vi "Agilent SNA Read Measurement.vi"(6 "Channel":i8=1 min=1 max=99 step=1, 7 "Agilent SNA & SWP":T2, 8 "error in (no error)":errorcluster, 11 "VISA Resource Names":T3) -> (0 "error out":errorcluster, 1 "Parameter":T1 {"Stimulus Port" min=1 step=1; "Response Port" min=1 step=1}, 2 "Measurement":T4=enum."Analog In - Aux In", 3 "dup VISA Resource Names":T3)   [LabVIEW 2011]
doc: "This VI for the HP 8753B is used to read the meausurement format.\n\n0 log magnitude\n1 phase\n2 delay\n3 Smith chart\n4 polar\n5 linear magnitude\n6 standing wave ratio\n7 real\n8 imaginary"
uses:
  TypeDefs/Agilent SNA Measurement.ctl
  TypeDefs/Agilent SNA VISA.ctl
  TypeDefs/Agilent SNA Instrument Info.ctl
  tests/S Parameter/TypeDefs/SP Parameter.ctl
panel:
  in  "Trace":i8=1 min=1 max=99 step=1
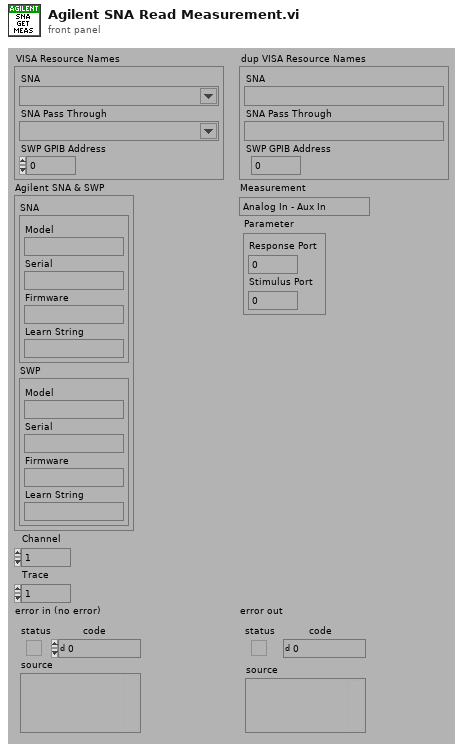
[diagram p1: front panel]
types:
  T1 = typedef "SP Parameter.ctl" = cluster{"Stimulus Port":i8, "Response Port":i8}
  T2 = typedef "Agilent SNA Instrument Info.ctl" = cluster{"SNA":cluster{"Model":string, "Serial":string, "Firmware":string, "Learn String":string}, "SWP":cluster{"Model":string, "Serial":string, "Firmware":string, "Learn String":string}}
  T3 = typedef "Agilent SNA VISA.ctl" = cluster{"SNA":refnum<visa-resource-name>, "SNA Pass Through":refnum<visa-resource-name>, "SWP GPIB Address":i32}
  T4 = typedef "Agilent SNA Measurement.ctl" = enum32{"SXX", "A", "B", "C", "R", "A/B", "A/C", "A/R", "B/A", "B/C", "B/R", "C/A", "C/B", "C/R", "R/A", "R/B", "R/C", "Analog In - Aux In"}
  T5 = typedef "Agilent SNA Model.ctl" = enum16{"Not Supported", "8757X"}
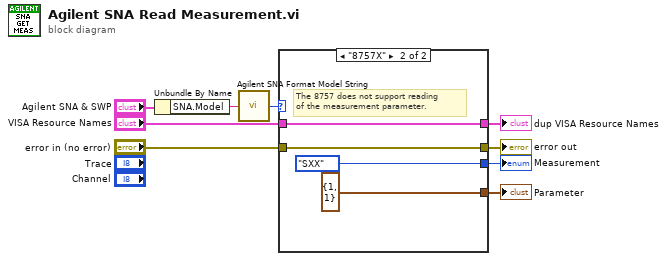
[diagram p0: block diagram]
diagram:
  n1 = Unbundle By Name("Agilent SNA & SWP") -> ("SNA.Model"=w2:string)
  n2 = call "Agilent SNA Format Model String.vi"("Model String"=w2) -> ("Model"=w4:T5)
  n3 = case shown="\"8757X\"" w4 {
    tunnel: "VISA Resource Names" -> [w10 w14]
    tunnel: "error in (no error)" -> [w11 w15]
    tunnel: [w11 w15] -> w7
    tunnel: [_ Agilent_SNA_Measurement."SXX" ("Display Format")] -> w6
    tunnel: [w10 w14] -> w5
    tunnel: [_ T1 {"Stimulus Port"=1, "Response Port"=1} ("Parameter")] -> w1
    frame "Not Supported" {
    }
    frame "8757X" {
      # "The 8757 does not support reading\nof the measurement parameter."
    }
  }
  "Measurement" <- w6
  "dup VISA Resource Names" <- w5
  "error out" <- w7
  "Parameter" <- w1
